vi "Read_Write_INI.vi"(2 "Section":string, 5 "Data_In":T1, 11 "Error_In":errorcluster, 13 "INI_Select":T3) -> (6 "Data_Out":T1, 15 "Error_Out":errorcluster)   [LabVIEW 2023]
doc: "Used to read and write the INI file."
uses:
  Controls/INI_Operation_Select.ctl
  Controls/INI_Data.ctl
  Controls/Total_Cash_Count.ctl
  <vilib>/Utility/config.llb/Read Key (String).vi
  <vilib>/Utility/config.llb/Write Key (String).vi
  <vilib>/Utility/config.llb/NI_LVConfig.lvlib
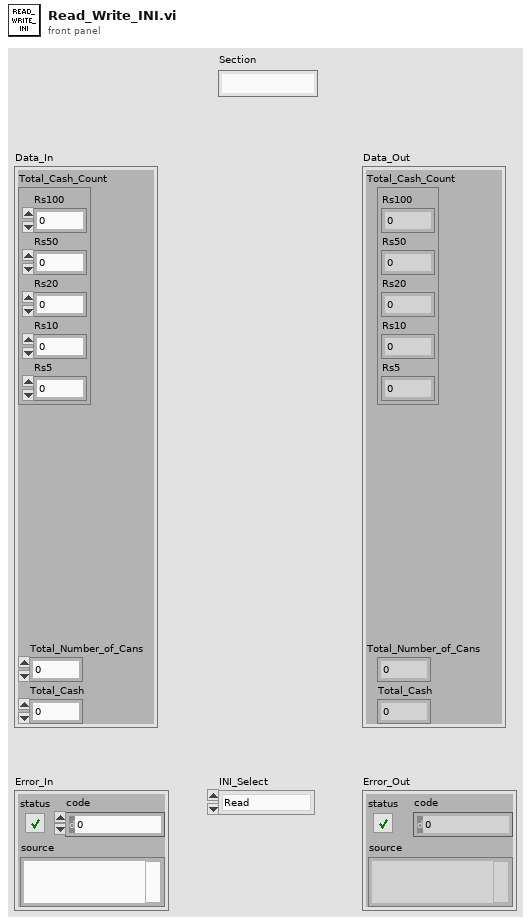
[diagram p1: front panel]
types:
  T1 = typedef "INI_Data.ctl" = cluster{"Total_Cash_Count":T2, "Total_Number_of_Cans":i32, "Total_Cash":i32}
  T2 = typedef "Total_Cash_Count.ctl" = cluster{"Rs100":i32, "Rs50":i32, "Rs20":i32, "Rs10":i32, "Rs5":i32}
  T3 = typedef "INI_Operation_Select.ctl" = enum16{"Read", "Write"}
  T4 = typedef "NI_LVConfig.lvlib/Config Data RefNum.ctl" = refnum<k1>
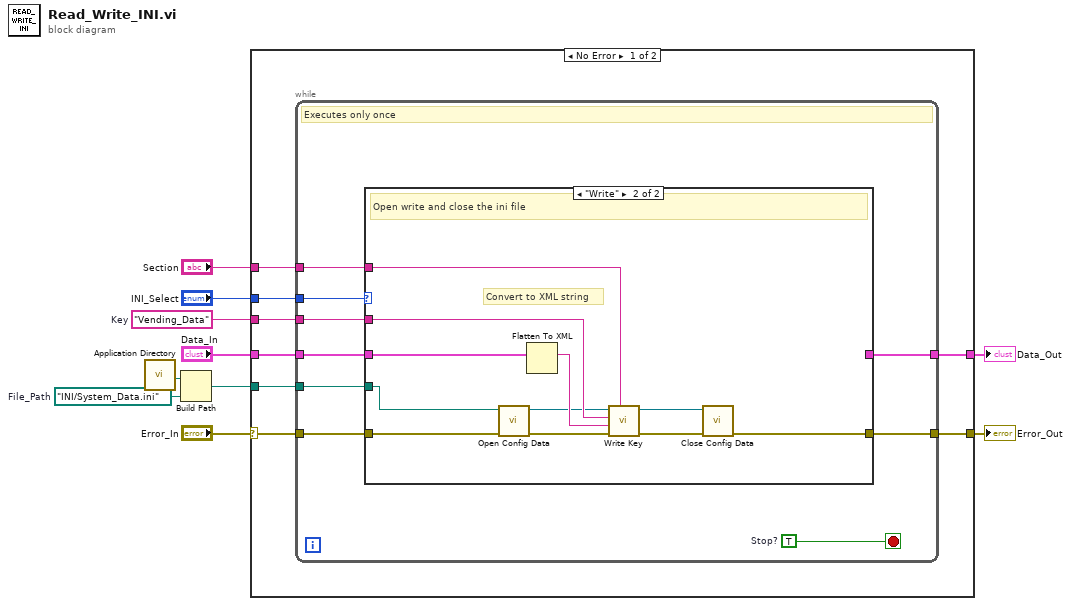
[diagram p0: block diagram]
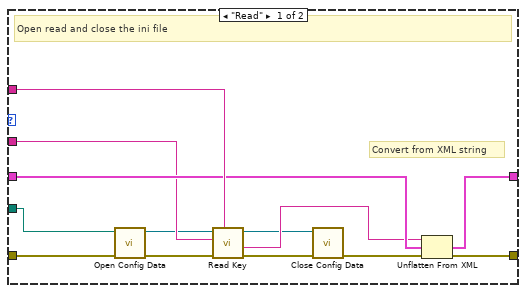
[diagram p2: hidden frame]
diagram:
  w2 = path "INI/System_Data.ini"  # File_Path
  w5 = "Vending_Data"  # Key
  n1 = call <vilib>:"Application Directory.vi"() -> ("Application Directory"=w3:path)
  n2 = Build Path(base path=w3, name or relative path=w2) -> (appended path=w1:path)
  n3 = case shown="No Error" "Error_In" {
    selector: "Error_In" -> [w11 w52]
    tunnel: [w18 w52] -> w10
    tunnel: w1 -> [w17 _]
    tunnel: "INI_Select" -> [w16 _]
    tunnel: "Section" -> [w15 _]
    tunnel: "Data_In" -> [w14 _]
    tunnel: [w13 _] -> w6
    tunnel: w5 -> [w12 _]
    frame No Error {
      n4 = while {
        tunnel: w11 -> [w27]
        tunnel: [w26] -> w18
        tunnel: w17 -> [w25]
        tunnel: w16 -> [w24]
        tunnel: w15 -> [w23]
        tunnel: w14 -> [w21]
        tunnel: [w20] -> w13
        tunnel: w12 -> [w19]
        stop <- w22 stop-if-true
        w22 = TRUE  # Stop?
        # "Executes only once"
        n5 = case shown="\"Write\"" w24 {
          tunnel: w27 -> [w34 w47]
          tunnel: [w35 w42] -> w26
          tunnel: w25 -> [w32 w44]
          tunnel: w23 -> [w40 w51]
          tunnel: w21 -> [w39 w50]
          tunnel: [w37 _] -> w20
          tunnel: w19 -> [w36 w48]
          frame "Read" {
            # "Convert from XML string"
            # "Open read and close the ini file"
            n6 = call <vilib>:"Open Config Data.vi"("error in (no error)"=w34, "configuration file path"=w32) -> ("error out"=w33:errorcluster, "refnum"=w31:T4)  [unwired: 7 in, 1 out]
            n7 = call-poly <vilib>:"Read Key.vi"("section"=w40, "error in (no error)"=w33, "key"=w36, "refnum"=w31) -> ("error out"=w30:errorcluster, "value"=w38:string, "refnum out"=w28:T4)  [unwired: 4 in, 1 out]
            n8 = call <vilib>:"Close Config Data.vi"("error in (no error)"=w30, "refnum"=w28) -> ("error out"=w29:errorcluster)  [unwired: 8 in, 1 out]
            n9 = Unflatten From XML(xml string=w38, type=w39, error in (no error)=w29) -> (value=w37:T1, error out=w35:errorcluster)
          }
          frame "Write" {
            # "Convert to XML string"
            # "Open write and close the ini file"
            n10 = call <vilib>:"Open Config Data.vi"("error in (no error)"=w47, "configuration file path"=w44) -> ("error out"=w45:errorcluster, "refnum"=w43:T4)  [unwired: 7 in, 1 out]
            n11 = Flatten To XML(6:w50) -> (2:w49:string)
            n12 = call-poly <vilib>:"Write Key.vi"("section"=w51, "error in (no error)"=w45, "value"=w49, "key"=w48, "refnum"=w43) -> ("error out"=w46:errorcluster, "refnum out"=w41:T4)  [unwired: 4 in, 1 out]
            n13 = call <vilib>:"Close Config Data.vi"("error in (no error)"=w46, "refnum"=w41) -> ("error out"=w42:errorcluster)  [unwired: 8 in, 1 out]
          }
        }
      }
    }
    frame Error {
    }
  }
  "Error_Out" <- w10
  "Data_Out" <- w6
